vi "SAOMM-FalconFixer_patched.vi"(0 "PRAMMS VRN":refnum<visa-resource-name>="COM4", 1 "ROIYOffset":u16, 2 "ROIXOffset":u16, 3 "Binning":u16(ring) items=["1 x 1"=1, "2 x 2"=2, "4 x 4"=4, "5 x 5"=5], 5 "command.ini":path=path "C:/BonOMM/Config/command.ini", 7 "Signature":u32, 11 "PRAMMS Error":errorcluster, 12 "ROIWidth":u16, 13 "ROIHeight":u16) -> (8 "Error":bool)   [LabVIEW 2019]
uses:
  EXTRACT-DATA-UINT32.vi
  Polymorphics/Num2littleEndian(U16).vi
  Polymorphics/Num2littleEndian(DBL).vi
panel:
  out "Errors Received":i32[](array[numeric])
  out "Initial Parameters Sent":bool
  out "Defaults Sent":bool
  out "Acquisition Stopped":bool
  out "Acquisition Started":bool
  out "Acknowledgement":i32
  in  "Pixel X":dbl
  in  "Pixel Y":dbl
  out "MessageType":cluster{string[], u32[]}
  out "DumpArray":string[](array[string])
  out "Actif":bool
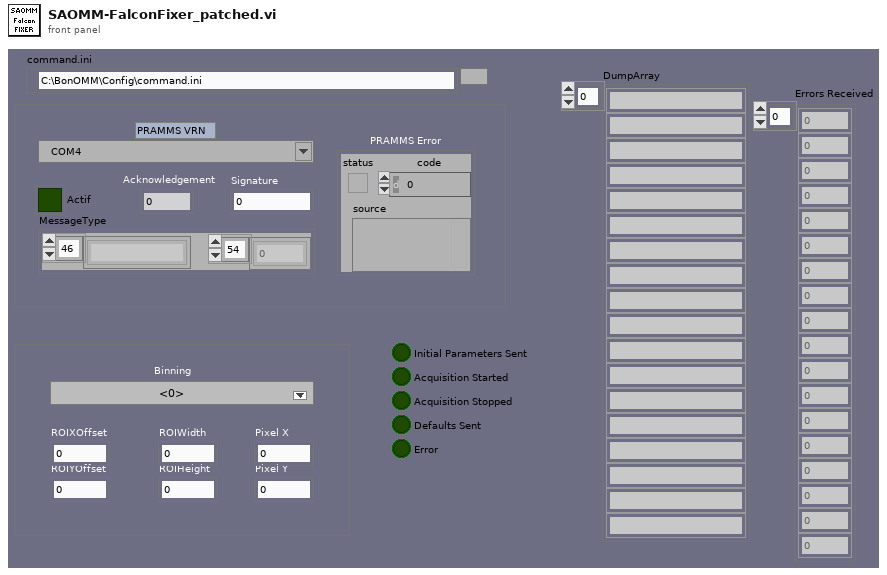
[diagram p1: front panel]
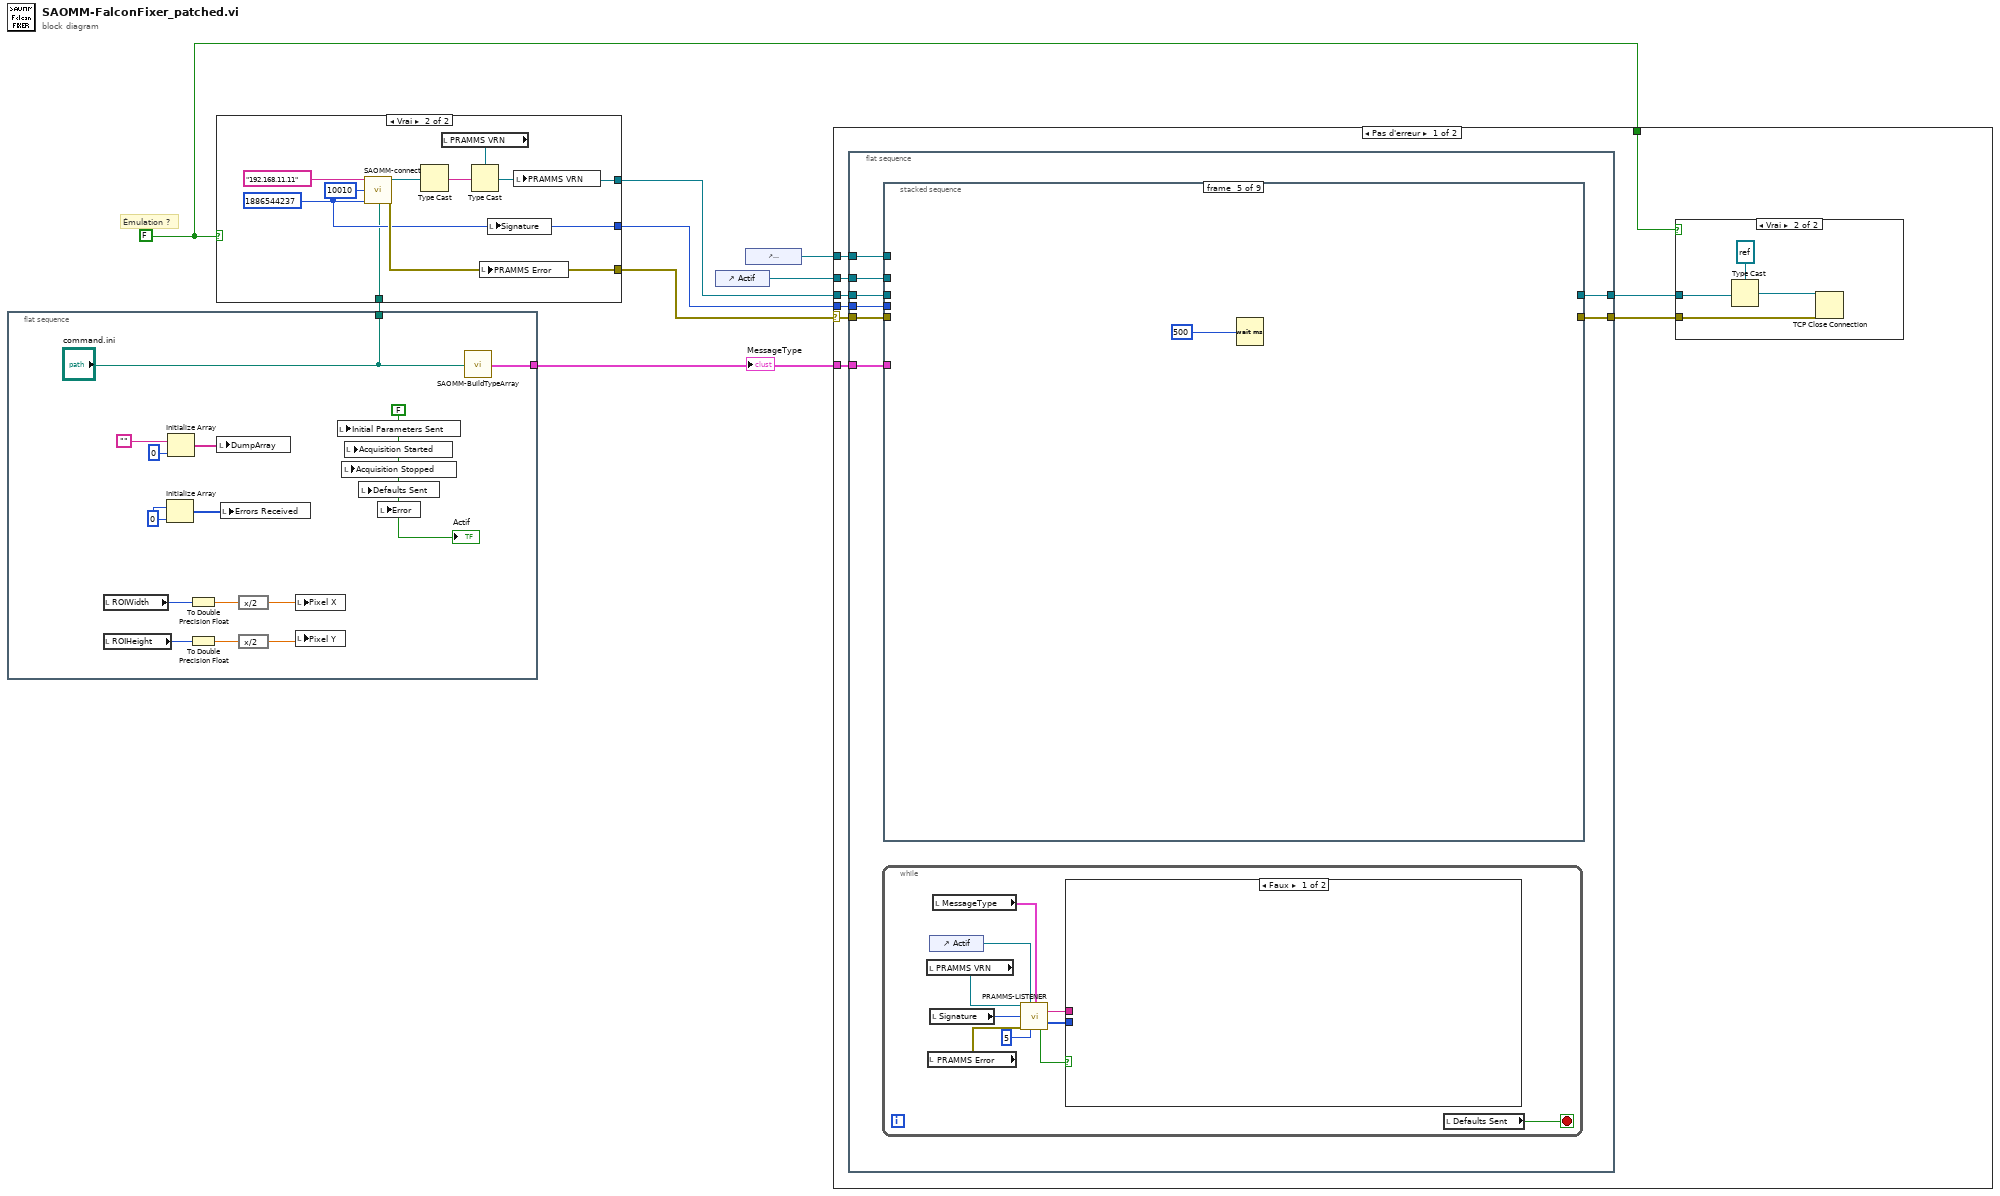
[diagram p0: block diagram]
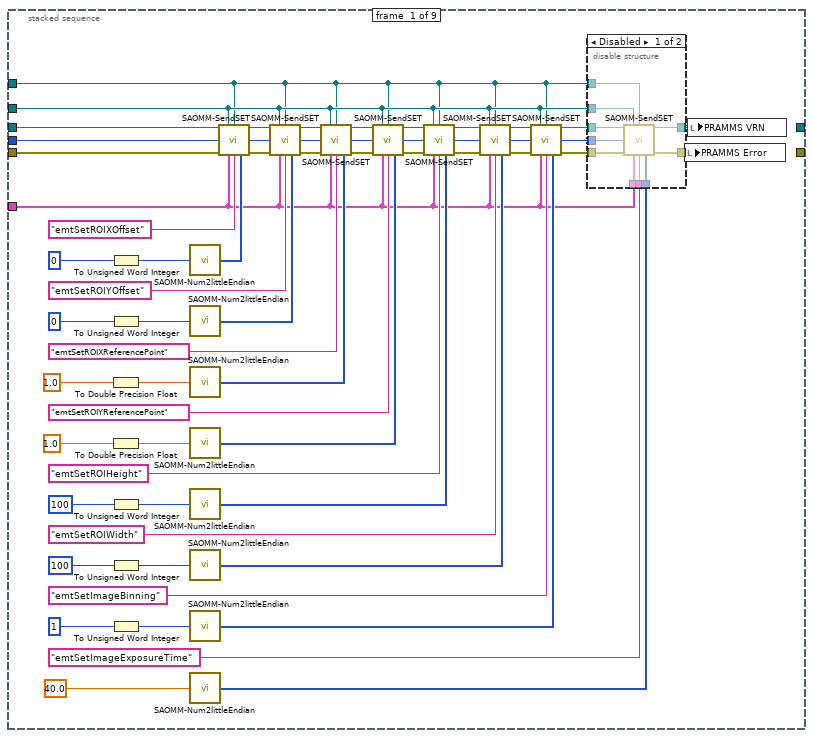
[diagram p3: hidden frame]
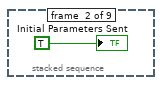
[diagram p5: hidden frame]
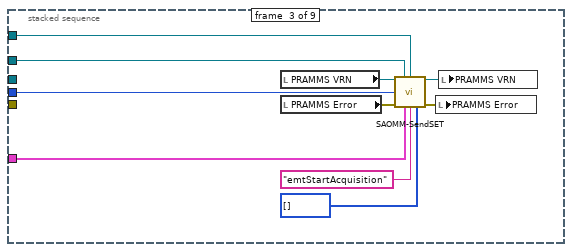
[diagram p6: hidden frame]
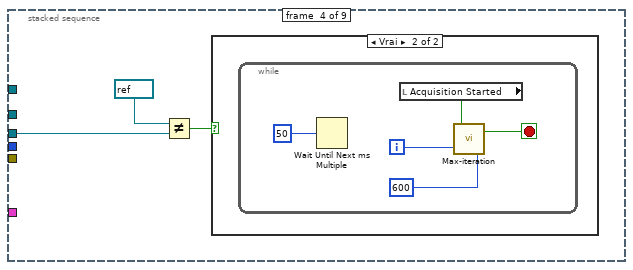
[diagram p7: hidden frame]
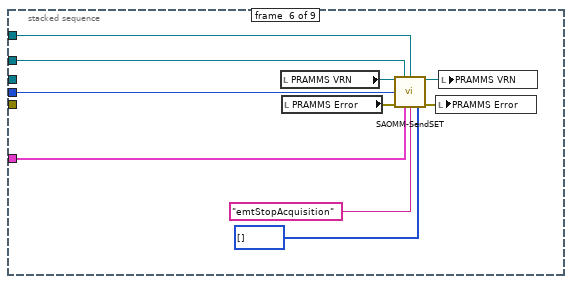
[diagram p9: hidden frame]
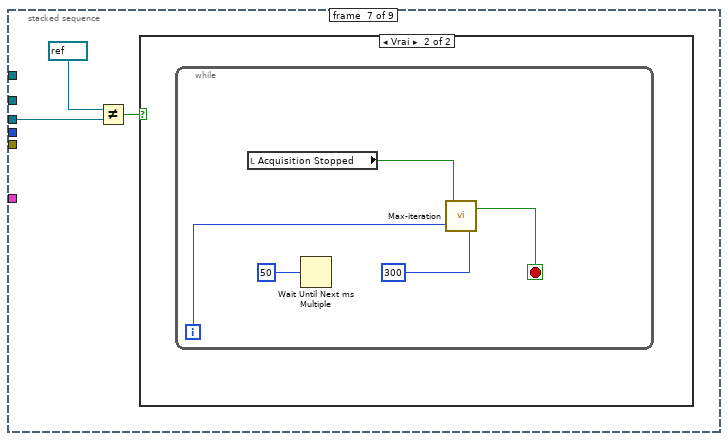
[diagram p10: hidden frame]
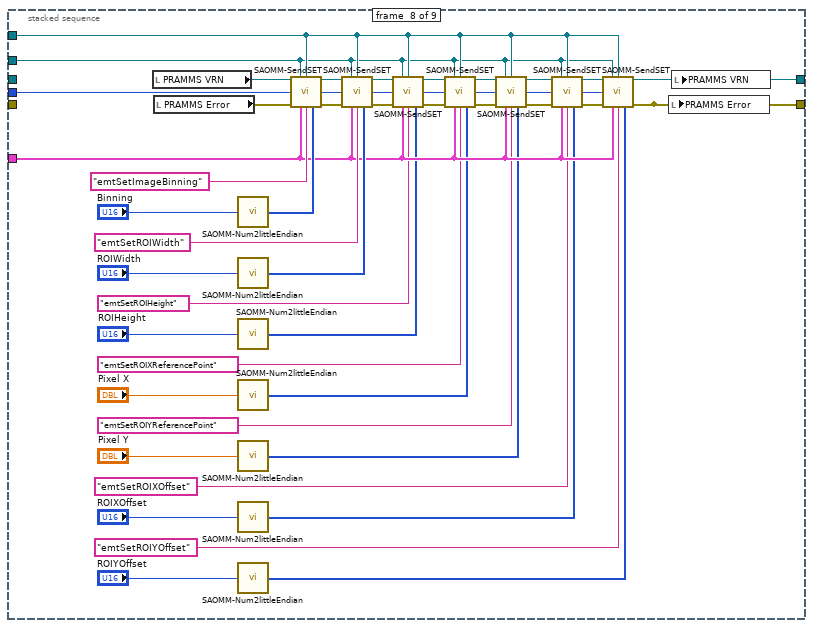
[diagram p12: hidden frame]
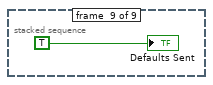
[diagram p13: hidden frame]
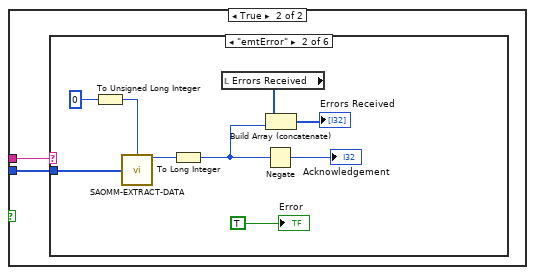
[diagram p14: hidden frame]
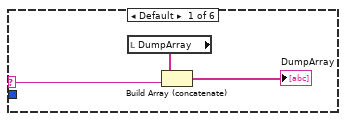
[diagram p15: hidden frame]
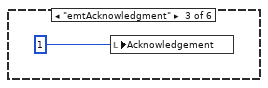
[diagram p16: hidden frame]
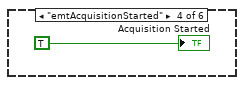
[diagram p17: hidden frame]
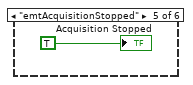
[diagram p18: hidden frame]
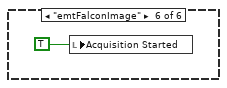
[diagram p19: hidden frame]
diagram:
  w2 = FALSE
  # "Émulation ?"
  n1 = flat-sequence {
    tunnel: [w22] -> w4
    tunnel: ["command.ini"] -> w1
    frame #0 {
      w18 = 0 ("dimension size")
      w12 = FALSE ("Initial Parameters Sent")
      n2 = local read "ROIWidth"() -> (w16:u16)
      n3 = local read "ROIHeight"() -> (w13:u16)
      n4 = Initialize Array(w18, w18) -> (w17:i32[])
      n5 = Initialize Array("", 0 ("dimension size")) -> (w19:string[])
      n6 = To Double Precision Float(number=w16) -> (double precision float=w15:dbl)
      n7 = To Double Precision Float(number=w13) -> (double precision float=w14:dbl)
      n8 = local write "DumpArray"(w19) -> ()
      n9 = local write "Errors Received"(w17) -> ()
      n10 = expression code="x/2"(w15) -> (w11:dbl)
      n11 = expression code="x/2"(w14) -> (w10:dbl)
      n12 = local write "Pixel X"(w11) -> ()
      n13 = local write "Pixel Y"(w10) -> ()
      n14 = local write "Initial Parameters Sent"(w12) -> ()
      n15 = local write "Acquisition Stopped"(w12) -> ()
      n16 = local write "Acquisition Started"(w12) -> ()
      n17 = local write "Defaults Sent"(w12) -> ()
      n18 = local write "Error"(w12) -> ()
      n19 = call "SAOMM-BuildTypeArray.vi"("command.ini"="command.ini") -> ("CommandArray"=w22:cluster{string[], u32[]})  [unwired: 14 in]
      "Actif" <- w12
    }
  }
  n20 = case shown="Vrai" w2 {
    tunnel: ["PRAMMS VRN" w27] -> w5
    tunnel: ["PRAMMS Error" w32] -> w3
    tunnel: ["Signature" w31] -> w6
    tunnel: w1 -> [_ w26]
    frame False {
    }
    frame True {
      w31 = u32 1886544237 ("Signature")
      n21 = call "SAOMM-connect.vi"("IP"="192.168.11.11", "Port"=u16 10010, "Signature"=w31, "Command.ini"=w26) -> ("connection ID"=w28:refnum<k5>, "Error OUT"=w32:errorcluster)  [unwired: 7 in, 3 out]
      n22 = Type Cast(x=w28) -> (*(type *) &x=w29:string)  [unwired: 1 in]
      n23 = local read "PRAMMS VRN"() -> (w30:refnum<visa-resource-name>)
      n24 = Type Cast(type=w30, x=w29) -> (*(type *) &x=w27:refnum<visa-resource-name>)
      n25 = local write "PRAMMS Error"(w32) -> ()
      n26 = local write "Signature"(w31) -> ()
      n27 = local write "PRAMMS VRN"(w27) -> ()
    }
  }
  n28 = control-ref of="Actif"() -> (w8:refnum<vi>)
  n29 = control-ref of="Acknowledgement"() -> (w7:refnum<vi>)
  n30 = case shown="Pas d'erreur" w3 {
    selector: w3 -> [w38 _]
    tunnel: w8 -> [w43 _]
    tunnel: w7 -> [w42 _]
    tunnel: w6 -> [w41 _]
    tunnel: w5 -> [w40 _]
    tunnel: w4 -> [w39 _]
    tunnel: w2 -> [w35 _]
    frame No Error {
      n31 = flat-sequence {
        tunnel: w39 -> [w55]
        tunnel: w43 -> [w54]
        tunnel: w42 -> [w53]
        tunnel: w38 -> [w52]
        tunnel: w41 -> [w51]
        tunnel: w40 -> [w50]
        tunnel: [w49] -> w36
        tunnel: [w48] -> w37
        frame #0 {
          n32 = while {
            stop <- w202 stop-if-true
            n33 = local read "PRAMMS VRN"() -> (w210:refnum<visa-resource-name>)
            n34 = local read "PRAMMS Error"() -> (w208:errorcluster)
            n35 = control-ref of="Actif"() -> (w207:refnum<vi>)
            n36 = local read "Signature"() -> (w209:u32)
            n37 = local read "MessageType"() -> (w206:cluster{string[], u32[]})
            n38 = call "PRAMMS-LISTENER.vi"("PRAMMS-COMM IN"=w210, "Bool Refnum"=w207, "MessageTypeArray"=w206, "Signature"=w209, "Error IN"=w208, "ReadTimeOut"=5) -> ("Type"=w204:string, "ByteArray"=w203:u8[], "Received?"=w201:bool)  [unwired: 4 in, 3 out]
            n39 = case shown="Faux" w201 {
              tunnel: w204 -> [_ w212]
              tunnel: w203 -> [_ w211]
              frame False {
              }
              frame True {
                n40 = case shown="\"emtError\"" w212 {
                  selector: w212 -> [w214 _ _ _ _ _]
                  tunnel: w211 -> [_ w222 _ _ _ _]
                  frame Default {
                    n41 = local read "DumpArray"() -> (w215:string[])
                    n42 = Build Array (concatenate)(w215, w214) -> (→"DumpArray":string[])
                  }
                  frame "emtError" {
                    n43 = To Unsigned Long Integer(number=u32 0) -> (unsigned 32bit integer=w223:u32)
                    n44 = call-poly "SAOMM-EXTRACT-DATA.vi"("UINT32"=w223, "Data"=w222) -> ("Value"=w219:u32)  [unwired: 10 in, 3 out]
                    n45 = To Long Integer(number=w219) -> (32bit integer=w216:i32)
                    n46 = local read "Errors Received"() -> (w218:i32[])
                    n47 = Negate(x=w216) -> (-x=→"Acknowledgement":i32)
                    n48 = Build Array (concatenate)(w218, w216) -> (→"Errors Received":i32[])
                    "Error" <- TRUE ("Error")
                  }
                  frame "emtAcknowledgment" {
                    n49 = local write "Acknowledgement"(1 ("PrAMS-ACK")) -> ()
                  }
                  frame "emtAcquisitionStarted" {
                    "Acquisition Started" <- TRUE ("Acquisition Started")
                  }
                  frame "emtAcquisitionStopped" {
                    "Acquisition Stopped" <- TRUE ("Acquisition Stopped")
                  }
                  frame "emtFalconImage" {
                    n50 = local write "Acquisition Started"(TRUE ("Acquisition Started")) -> ()
                  }
                }
              }
            }
            n51 = local read "Defaults Sent"() -> (w202:bool)
          }
          n52 = stacked-sequence {
            tunnel: w55 -> [w64 _ w130 _ _ w149 _ w180 _]
            tunnel: w54 -> [w60 _ w129 _ _ w148 _ w181 _]
            tunnel: w53 -> [w59 _ w128 _ _ w147 _ w182 _]
            tunnel: w52 -> [w86 _ _ _ _ _ _ _ _]
            tunnel: w51 -> [w61 _ w131 _ _ w150 _ w183 _]
            tunnel: w50 -> [w85 _ _ w132 _ _ w153 _ _]
            tunnel: [_ _ _ _ _ _ _ w160 _] -> w49
            tunnel: [_ _ _ _ _ _ _ w159 _] -> w48
            frame #0 {
              n53 = To Unsigned Word Integer(number=u16 0) -> (unsigned 16bit integer=w91:u16)
              n54 = To Unsigned Word Integer(number=u16 0) -> (unsigned 16bit integer=w90:u16)
              n55 = To Double Precision Float(number=1.0) -> (double precision float=w77:dbl)
              n56 = To Double Precision Float(number=1.0) -> (double precision float=w89:dbl)
              n57 = To Unsigned Word Integer(number=u16 100) -> (unsigned 16bit integer=w78:u16)
              n58 = To Unsigned Word Integer(number=u16 100) -> (unsigned 16bit integer=w88:u16)
              n59 = To Unsigned Word Integer(number=u16 1) -> (unsigned 16bit integer=w87:u16)
              n60 = call-poly "SAOMM-Num2littleEndian.vi"("Number"=w91) -> ("LiitleEndianedData"=w102:u8[])  [unwired: 14 in]
              n61 = call-poly "SAOMM-Num2littleEndian.vi"("Number"=w90) -> ("LiitleEndianedData"=w101:u8[])  [unwired: 14 in]
              n62 = call-poly "SAOMM-Num2littleEndian.vi"("Number"=w77) -> ("LiitleEndianedData"=w76:u8[])  [unwired: 14 in]
              n63 = call-poly "SAOMM-Num2littleEndian.vi"("Number"=w89) -> ("LiitleEndianedData"=w75:u8[])  [unwired: 14 in]
              n64 = call-poly "SAOMM-Num2littleEndian.vi"("Number"=w78) -> ("LiitleEndianedData"=w74:u8[])  [unwired: 14 in]
              n65 = call-poly "SAOMM-Num2littleEndian.vi"("Number"=w88) -> ("LiitleEndianedData"=w73:u8[])  [unwired: 14 in]
              n66 = call-poly "SAOMM-Num2littleEndian.vi"("Number"=w87) -> ("LiitleEndianedData"=w72:u8[])  [unwired: 14 in]
              n67 = call-poly "SAOMM-Num2littleEndian.vi"("Number"=40.0) -> ("LiitleEndianedData"=w62:u8[])  [unwired: 14 in]
              n68 = call "SAOMM-SendSET.vi"("PRAMMS-COMM IN"=w85, "Active Refnum"=w60, "PrAMS-ACK"=w59, "Signature"=w61, "Error IN"=w86, "MessageType"=w64, "Active SET"="emtSetROIXOffset", "Value (little endianed byte array)"=w102) -> ("PRAMMS-COMM OUT"=w95:refnum<visa-resource-name>, "Error OUT"=w96:errorcluster)  [unwired: 4 in, 2 out]
              n69 = call "SAOMM-SendSET.vi"("PRAMMS-COMM IN"=w95, "Active Refnum"=w60, "PrAMS-ACK"=w59, "Signature"=w61, "Error IN"=w96, "MessageType"=w64, "Active SET"="emtSetROIYOffset", "Value (little endianed byte array)"=w101) -> ("PRAMMS-COMM OUT"=w94:refnum<visa-resource-name>, "Error OUT"=w97:errorcluster)  [unwired: 4 in, 2 out]
              n70 = call "SAOMM-SendSET.vi"("PRAMMS-COMM IN"=w94, "Active Refnum"=w60, "PrAMS-ACK"=w59, "Signature"=w61, "Error IN"=w97, "MessageType"=w64, "Active SET"="emtSetROIXReferencePoint", "Value (little endianed byte array)"=w76) -> ("PRAMMS-COMM OUT"=w93:refnum<visa-resource-name>, "Error OUT"=w98:errorcluster)  [unwired: 4 in, 2 out]
              n71 = call "SAOMM-SendSET.vi"("PRAMMS-COMM IN"=w93, "Active Refnum"=w60, "PrAMS-ACK"=w59, "Signature"=w61, "Error IN"=w98, "MessageType"=w64, "Active SET"="emtSetROIYReferencePoint", "Value (little endianed byte array)"=w75) -> ("PRAMMS-COMM OUT"=w92:refnum<visa-resource-name>, "Error OUT"=w99:errorcluster)  [unwired: 4 in, 2 out]
              n72 = call "SAOMM-SendSET.vi"("PRAMMS-COMM IN"=w92, "Active Refnum"=w60, "PrAMS-ACK"=w59, "Signature"=w61, "Error IN"=w99, "MessageType"=w64, "Active SET"="emtSetROIHeight", "Value (little endianed byte array)"=w74) -> ("PRAMMS-COMM OUT"=w84:refnum<visa-resource-name>, "Error OUT"=w83:errorcluster)  [unwired: 4 in, 2 out]
              n73 = call "SAOMM-SendSET.vi"("PRAMMS-COMM IN"=w84, "Active Refnum"=w60, "PrAMS-ACK"=w59, "Signature"=w61, "Error IN"=w83, "MessageType"=w64, "Active SET"="emtSetROIWidth", "Value (little endianed byte array)"=w73) -> ("PRAMMS-COMM OUT"=w81:refnum<visa-resource-name>, "Error OUT"=w82:errorcluster)  [unwired: 4 in, 2 out]
              n74 = call "SAOMM-SendSET.vi"("PRAMMS-COMM IN"=w81, "Active Refnum"=w60, "PrAMS-ACK"=w59, "Signature"=w61, "Error IN"=w82, "MessageType"=w64, "Active SET"="emtSetImageBinning", "Value (little endianed byte array)"=w72) -> ("PRAMMS-COMM OUT"=w66:refnum<visa-resource-name>, "Error OUT"=w65:errorcluster)  [unwired: 4 in, 2 out]
              n75 = disable-structure shown="Disabled" {
                disable-tunnel: w66 -> [w118 w120]
                disable-tunnel: w65 -> [w117 w119]
                disable-tunnel: w64 -> [w116 _]
                disable-tunnel: "emtSetImageExposureTime" -> [w115 _]
                disable-tunnel: w62 -> [w114 _]
                disable-tunnel: w61 -> [w113 _]
                disable-tunnel: w60 -> [w112 _]
                disable-tunnel: w59 -> [w111 _]
                disable-tunnel: [w110 w120] -> w58
                disable-tunnel: [w109 w119] -> w57
                frame Disabled {
                  n76 = call "SAOMM-SendSET.vi"("PRAMMS-COMM IN"=w118, "Active Refnum"=w112, "PrAMS-ACK"=w111, "Signature"=w113, "Error IN"=w117, "MessageType"=w116, "Active SET"=w115, "Value (little endianed byte array)"=w114) -> ("PRAMMS-COMM OUT"=w110:refnum<visa-resource-name>, "Error OUT"=w109:errorcluster)  [unwired: 4 in, 2 out]
                }
                frame Enabled {
                }
              }
              n77 = local write "PRAMMS Error"(w57) -> ()
              n78 = local write "PRAMMS VRN"(w58) -> ()
            }
            frame #1 {
              "Initial Parameters Sent" <- TRUE
            }
            frame #2 {
              n79 = local read "PRAMMS VRN"() -> (w125:refnum<visa-resource-name>)
              n80 = local read "PRAMMS Error"() -> (w124:errorcluster)
              n81 = call "SAOMM-SendSET.vi"("PRAMMS-COMM IN"=w125, "Active Refnum"=w129, "PrAMS-ACK"=w128, "Signature"=w131, "Error IN"=w124, "MessageType"=w130, "Active SET"="emtStartAcquisition", "Value (little endianed byte array)"=u8[] []) -> ("PRAMMS-COMM OUT"=w123:refnum<visa-resource-name>, "Error OUT"=w122:errorcluster)  [unwired: 4 in, 2 out]
              n82 = local write "PRAMMS Error"(w122) -> ()
              n83 = local write "PRAMMS VRN"(w123) -> ()
            }
            frame #3 {
              n84 = Not Equal?(x=refnum<visa-resource-name> "-1", y=w132) -> (x != y?=w133:bool)
              n85 = case shown="Vrai" w133 {
                frame False {
                }
                frame True {
                  n86 = while {
                    i -> [w137]
                    stop <- w136 stop-if-true
                    n87 = Wait Until Next ms Multiple(millisecond multiple=u32 50) -> ()  [unwired: 1 out]
                    n88 = local read "Acquisition Started"() -> (w138:bool)
                    n89 = call "Max-iteration.vi"("i max"=600, "i act"=w137, "Valeur entrante"=w138) -> ("break ?"=w136:bool)
                  }
                }
              }
            }
            frame #4 {
              n90 = Wait (ms)(milliseconds to wait=u32 500) -> ()  [unwired: 1 out]
            }
            frame #5 {
              n91 = local read "PRAMMS VRN"() -> (w144:refnum<visa-resource-name>)
              n92 = local read "PRAMMS Error"() -> (w143:errorcluster)
              n93 = call "SAOMM-SendSET.vi"("PRAMMS-COMM IN"=w144, "Active Refnum"=w148, "PrAMS-ACK"=w147, "Signature"=w150, "Error IN"=w143, "MessageType"=w149, "Active SET"="emtStopAcquisition", "Value (little endianed byte array)"=u8[] []) -> ("PRAMMS-COMM OUT"=w142:refnum<visa-resource-name>, "Error OUT"=w141:errorcluster)  [unwired: 4 in, 2 out]
              n94 = local write "PRAMMS Error"(w141) -> ()
              n95 = local write "PRAMMS VRN"(w142) -> ()
            }
            frame #6 {
              n96 = Not Equal?(x=refnum<visa-resource-name> "-1", y=w153) -> (x != y?=w151:bool)
              n97 = case shown="Vrai" w151 {
                frame False {
                }
                frame True {
                  n98 = while {
                    i -> [w155]
                    stop <- w154 stop-if-true
                    n99 = local read "Acquisition Stopped"() -> (w156:bool)
                    n100 = Wait Until Next ms Multiple(millisecond multiple=u32 50) -> ()  [unwired: 1 out]
                    n101 = call "Max-iteration.vi"("i max"=300, "i act"=w155, "Valeur entrante"=w156) -> ("break ?"=w154:bool)
                  }
                }
              }
            }
            frame #7 {
              n102 = local read "PRAMMS VRN"() -> (w169:refnum<visa-resource-name>)
              n103 = local read "PRAMMS Error"() -> (w168:errorcluster)
              n104 = call-poly "SAOMM-Num2littleEndian.vi"("Number"="Binning") -> ("LiitleEndianedData"=w198:u8[])  [unwired: 14 in]
              n105 = call-poly "SAOMM-Num2littleEndian.vi"("Number"="ROIWidth") -> ("LiitleEndianedData"=w197:u8[])  [unwired: 14 in]
              n106 = call-poly "SAOMM-Num2littleEndian.vi"("Number"="ROIHeight") -> ("LiitleEndianedData"=w179:u8[])  [unwired: 14 in]
              n107 = call-poly "SAOMM-Num2littleEndian.vi"("Number"="Pixel X") -> ("LiitleEndianedData"=w178:u8[])  [unwired: 14 in]
              n108 = call-poly "SAOMM-Num2littleEndian.vi"("Number"="Pixel Y") -> ("LiitleEndianedData"=w177:u8[])  [unwired: 14 in]
              n109 = call-poly "SAOMM-Num2littleEndian.vi"("Number"="ROIXOffset") -> ("LiitleEndianedData"=w176:u8[])  [unwired: 14 in]
              n110 = call-poly "SAOMM-Num2littleEndian.vi"("Number"="ROIYOffset") -> ("LiitleEndianedData"=w175:u8[])  [unwired: 14 in]
              n111 = call "SAOMM-SendSET.vi"("PRAMMS-COMM IN"=w169, "Active Refnum"=w181, "PrAMS-ACK"=w182, "Signature"=w183, "Error IN"=w168, "MessageType"=w180, "Active SET"="emtSetImageBinning", "Value (little endianed byte array)"=w198) -> ("PRAMMS-COMM OUT"=w191:refnum<visa-resource-name>, "Error OUT"=w192:errorcluster)  [unwired: 4 in, 2 out]
              n112 = call "SAOMM-SendSET.vi"("PRAMMS-COMM IN"=w191, "Active Refnum"=w181, "PrAMS-ACK"=w182, "Signature"=w183, "Error IN"=w192, "MessageType"=w180, "Active SET"="emtSetROIWidth", "Value (little endianed byte array)"=w197) -> ("PRAMMS-COMM OUT"=w190:refnum<visa-resource-name>, "Error OUT"=w193:errorcluster)  [unwired: 4 in, 2 out]
              n113 = call "SAOMM-SendSET.vi"("PRAMMS-COMM IN"=w190, "Active Refnum"=w181, "PrAMS-ACK"=w182, "Signature"=w183, "Error IN"=w193, "MessageType"=w180, "Active SET"="emtSetROIHeight", "Value (little endianed byte array)"=w179) -> ("PRAMMS-COMM OUT"=w189:refnum<visa-resource-name>, "Error OUT"=w194:errorcluster)  [unwired: 4 in, 2 out]
              n114 = call "SAOMM-SendSET.vi"("PRAMMS-COMM IN"=w189, "Active Refnum"=w181, "PrAMS-ACK"=w182, "Signature"=w183, "Error IN"=w194, "MessageType"=w180, "Active SET"="emtSetROIXReferencePoint", "Value (little endianed byte array)"=w178) -> ("PRAMMS-COMM OUT"=w188:refnum<visa-resource-name>, "Error OUT"=w195:errorcluster)  [unwired: 4 in, 2 out]
              n115 = call "SAOMM-SendSET.vi"("PRAMMS-COMM IN"=w188, "Active Refnum"=w181, "PrAMS-ACK"=w182, "Signature"=w183, "Error IN"=w195, "MessageType"=w180, "Active SET"="emtSetROIYReferencePoint", "Value (little endianed byte array)"=w177) -> ("PRAMMS-COMM OUT"=w187:refnum<visa-resource-name>, "Error OUT"=w186:errorcluster)  [unwired: 4 in, 2 out]
              n116 = call "SAOMM-SendSET.vi"("PRAMMS-COMM IN"=w187, "Active Refnum"=w181, "PrAMS-ACK"=w182, "Signature"=w183, "Error IN"=w186, "MessageType"=w180, "Active SET"="emtSetROIXOffset", "Value (little endianed byte array)"=w176) -> ("PRAMMS-COMM OUT"=w184:refnum<visa-resource-name>, "Error OUT"=w185:errorcluster)  [unwired: 4 in, 2 out]
              n117 = call "SAOMM-SendSET.vi"("PRAMMS-COMM IN"=w184, "Active Refnum"=w181, "PrAMS-ACK"=w182, "Signature"=w183, "Error IN"=w185, "MessageType"=w180, "Active SET"="emtSetROIYOffset", "Value (little endianed byte array)"=w175) -> ("PRAMMS-COMM OUT"=w160:refnum<visa-resource-name>, "Error OUT"=w159:errorcluster)  [unwired: 4 in, 2 out]
              n118 = local write "PRAMMS Error"(w159) -> ()
              n119 = local write "PRAMMS VRN"(w160) -> ()
            }
            frame #8 {
              "Defaults Sent" <- TRUE ("Defaults Sent")
            }
          }
        }
      }
      n120 = case shown="Vrai" w35 {
        tunnel: w37 -> [_ w44]
        tunnel: w36 -> [_ w47]
        frame False {
        }
        frame True {
          n121 = Type Cast(type=refnum<k5> refnum ("connection ID"), x=w47) -> (*(type *) &x=w46:refnum<k5>)
          n122 = TCP Close Connection(connection ID=w46, error in (no error)=w44) -> ()  [unwired: 1 in, 2 out]
        }
      }
    }
    frame Error {
    }
  }
  "MessageType" <- w4
